vi "init access point wireless.vi"(4 "radio2_pipe_count":u8, 5 "radio1_pipe_count":u8, 6 "device_rx_address_high_order_bytes_B":u32, 7 "device_rx_address_high_order_bytes_A":u32, 9 "wireless_channel_2":u8, 10 "wireless_channel_1":u8, 11 "ap_handle":u32) -> (2 "function return":i32, 3 "ap_handle out":u32)   [LabVIEW 2019, in "apdm.lvlib"]
doc: "APDM_EXPORT int apdm_init_access_point_wireless(apdm_ap_handle_t ap_handle,\n const uint8_t wireless_channel_1, const uint8_t wireless_channel_2,\n const uint32_t device_rx_address_high_order_bytes_A,\n const uint32_t device_rx_address_high_order_bytes_B,\n const uint8_t radio1_pipe_count, const uint8_t radio2_pipe_count);"
uses:
  apdm.lvlib
  Lee Lab/CP FES Walking 2018/Code/Working/LabVIEW/apdm.dll
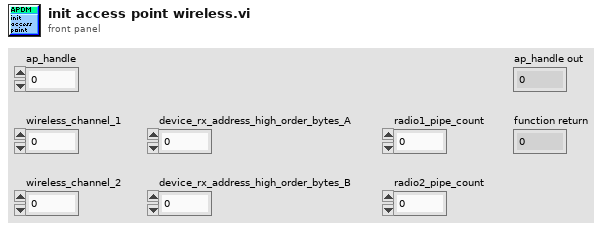
[diagram p1: front panel]
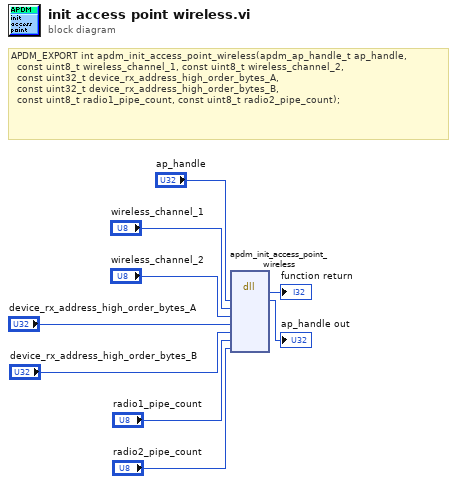
[diagram p0: block diagram]
diagram:
  # "APDM_EXPORT int apdm_init_access_point_wireless(apdm_ap_handle_t ap_handle,\n\t\tconst uint8_t wireless_channel_1, const uint8_t wireless_channel_2,\n\t\tconst uint32_t device_rx_address_high_order_bytes_A,\n\t\tconst uint32_t device_rx_address_high_order_bytes_B,\n\t\tconst uint8_t radio1_pipe_count, const uint8_t radio2_pipe_count);"
  n1 = dll-call lib="C:/Users/jfalesi/Dropbox/Lee Lab/CP FES Walking 2018/Code/Working/LabVIEW/apdm.*" fn="apdm_init_access_point_wireless"("ap_handle"="ap_handle", "wireless_channel_1"="wireless_channel_1", "wireless_channel_2"="wireless_channel_2", "device_rx_address_high_order_bytes_A"="device_rx_address_high_order_bytes_A", "device_rx_address_high_order_bytes_B"="device_rx_address_high_order_bytes_B", "radio1_pipe_count"="radio1_pipe_count", "radio2_pipe_count"="radio2_pipe_count") -> (→"function return":i32, "ap_handle"=→"ap_handle out":u32)  [unwired: 9 in, 2 out]
